vi "goToAngle.vi"(10 "gyro":dbl=-0.46 format="%.2f") -> (2 "x2":dbl=0.003082 format="%.2f")   [LabVIEW 2020]
uses:
  Robot Global Data.vi
  <vilib>/addons/control/pid/pid.llb/PID (DBL).vi
  <vilib>/addons/control/pid/NI_PID_pid.lvlib
panel:
  in  "invert":dbl=1.0
  in  "PID gains":T1={"proportional gain (Kc)"=0.0067, "integral time (Ti, min)"=0.0, "derivative time (Td, min)"=0.0} {"derivative time (Td, min)" format="%.3f"; "integral time (Ti, min)" format="%.20f"; "proportional gain (Kc)" format="%.20f"}
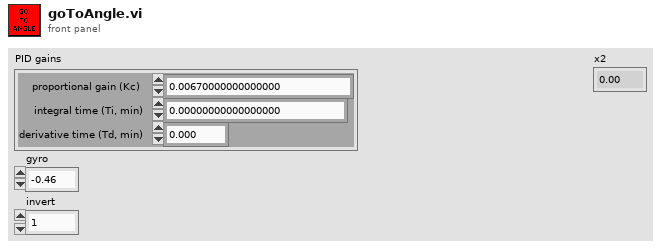
[diagram p1: front panel]
types:
  T1 = cluster{"proportional gain (Kc)":dbl, "integral time (Ti, min)":dbl, "derivative time (Td, min)":dbl}
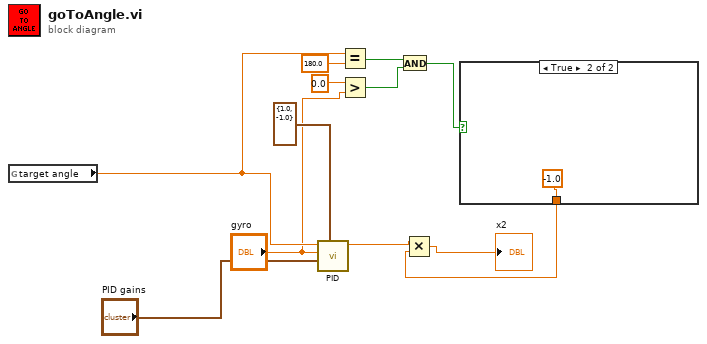
[diagram p0: block diagram]
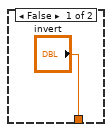
[diagram p2: hidden frame]
diagram:
  n1 = global read "Robot Global Data.vi" "target angle"() -> (w8:dbl)
  n2 = call-poly <vilib>:"PID.vi"("output range"=cluster{"output high":dbl, "output low":dbl} {"output high"=1.0, "output low"=-1.0}, "PID gains"="PID gains", "process variable"="gyro", "setpoint"=w8) -> ("output"=w9:dbl)  [unwired: 6 in, 1 out]
  n3 = Equal?(x=w8, y=180.0) -> (x = y?=w6:bool)
  n4 = Greater?(x=0.0 ("y"), y="gyro") -> (0:w5:bool)
  n5 = And(x=w6, y=w5) -> (x .and. y?=w4:bool)
  n6 = case shown="True" w4 {
    tunnel: ["invert" -1.0 ("invert")] -> w3
    frame False {
    }
    frame True {
    }
  }
  n7 = Multiply(x=w9, y=w3) -> (x*y=→"x2":dbl)
